vi "PrefDialog-old.vi"(8 "error in (no error)":errorcluster, 11 "MyPluginsBase in":refnum<class "NHRGridSim.lvclass">) -> (0 "error out":errorcluster, 1 "Save As":bool, 2 "Changed":bool, 3 "MyPluginsBase out":refnum<class "NHRGridSim.lvclass">)   [LabVIEW 2018, in "AcPwrPlugins.lvlib" / "NHRGridSim.lvclass"]
doc: "This VI opens up the modal preference dialog window and allows a user to configure the properties with new values, or keep the existing values from the last time the function was called. The user can also save the new values to a new file name and new type name using the save as button."
uses:
  NHRGridSim.lvclass
  C:/Program Files (x86)/National Instruments/LabVIEW 2018/user.lib/NIST/BaseClasses/BasePlugin_class/BasePlugin.lvclass
  C:/Users/Public/Projects/ICDAS/NistPluggableModules/AcPwr/AcPwrPlugins/AcPwrBaseClass/AcPwrBase.lvclass
  TypeDefs/Device(s)Settings.ctl
  TypeDefs/Modules.ctl
  Measurements.ctl
  TypeDefs/MeasurementType.ctl
  <userlib>/NIST/BaseClasses/BasePlugin_class/BasePlugin.lvclass/BasePlugin.ctl
  AcPwrBaseClass/AcPwrBase.lvclass/AcPwrBase.ctl
  <userlib>/NIST/BaseClasses/BasePlugin_class/Accessors/Read PluginIniFilePath.vi
  AcPwrBaseClass/Accessors/Read BaseConfig.vi
  AcPwrBaseClass/Accessors/Read BaseMeasurements.vi
  <userlib>/NIST/BaseClasses/BasePlugin_class/Accessors/Write PluginIniFilePath.vi
  <vilib>/Utility/config.llb/NI_LVConfig.lvlib
  AcPwrBaseClass/AcPwrBase.lvclass
panel:
  in  "Measurements":T1 {"Phase" items=["All", "A Phase", "B Phase", "C Phase"]}
  in  "Device(s)Settings":T3 {"Modules"."Phase (0: All)" items=["All", "A Phase", "B Phase", "C Phase"]; "Modules"."Mode" items=["3-Phase AC", "AC", "DC", "AC - AC - AC", "DC - DC - DC", "2-Phase AC - AC", "2-Phase AC - DC", "AC - AC", "AC - DC", "AC - AC - DC", "AC - DC - DC", "DC - AC", "DC - DC", "AC - DC - AC", "DC - AC - AC", "DC - AC - DC"]}
  in  "btnSaveAs":bool
  in  "Measurement RefreshTime (ms)":u32
  in  "btnSave":bool
  in  "btnCancel":bool
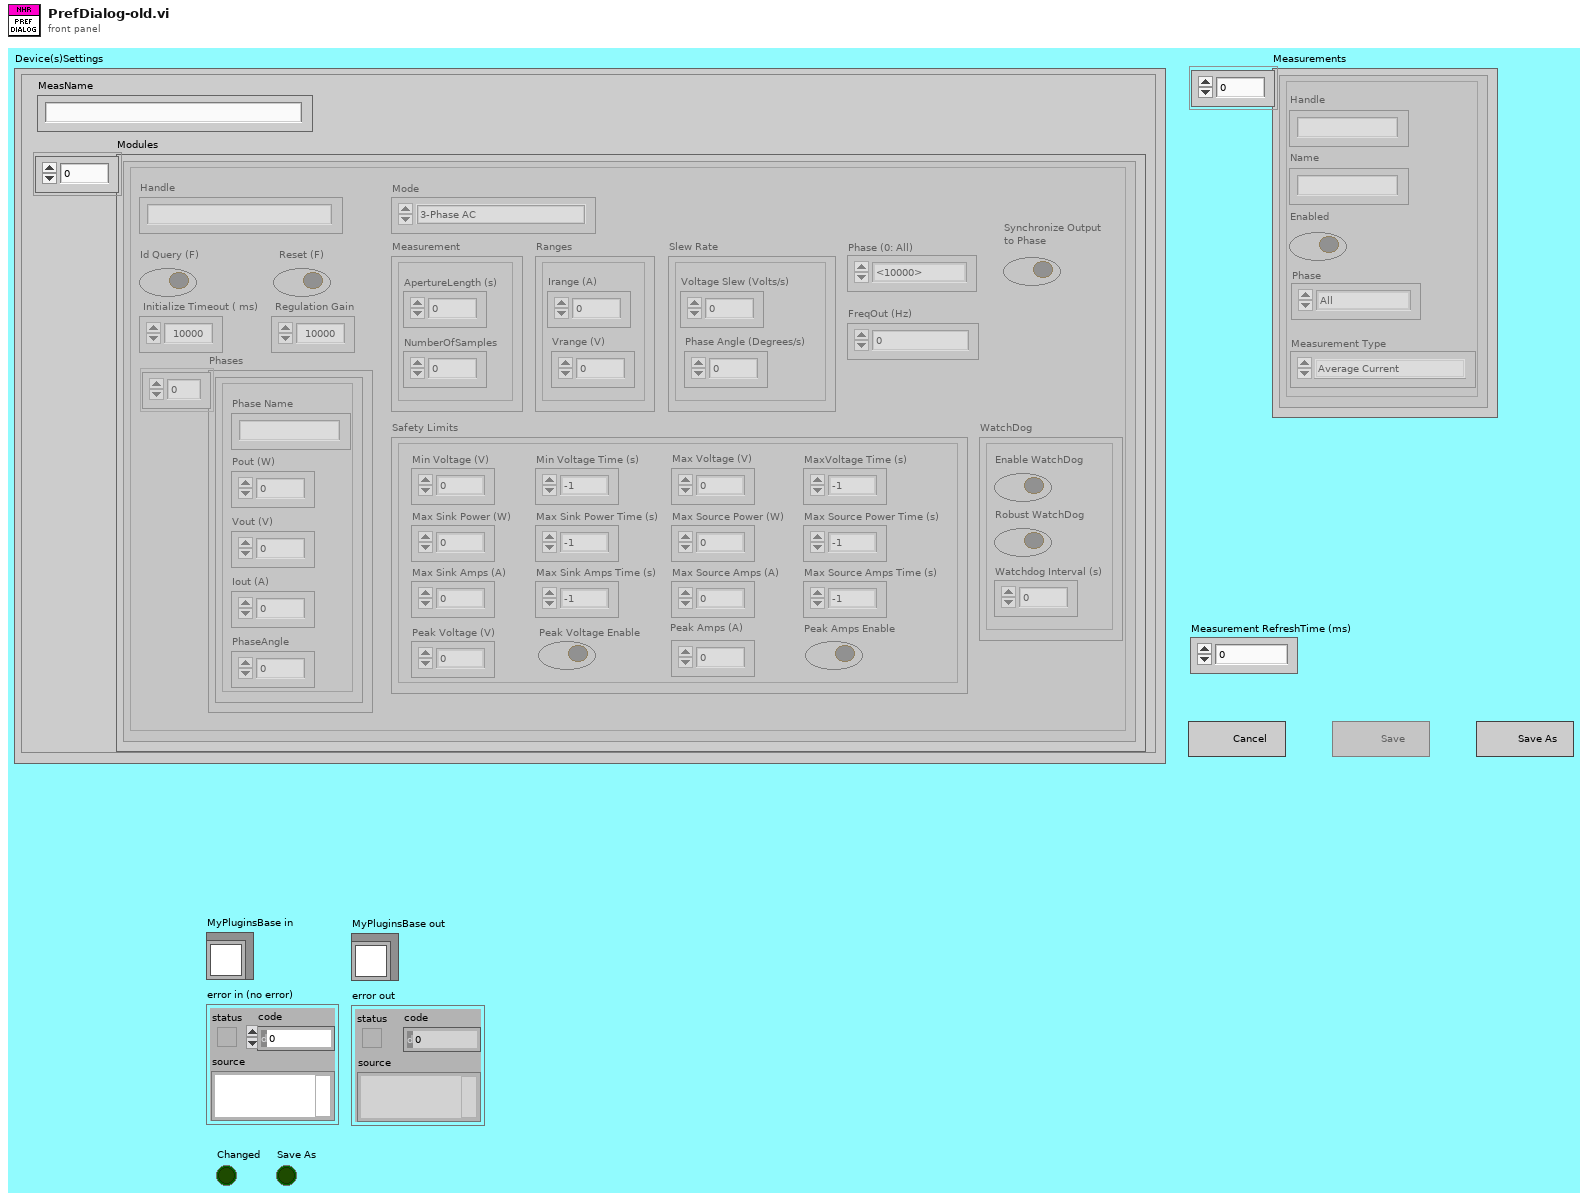
[diagram p1: front panel]
types:
  T1 = typedef "AcPwrPlugins.lvlib/NHRGridSim.lvclass/Measurements.ctl" = cluster{"Handle":string, "Name":string, "Enabled ":bool, "Measurement Value":dbl, "Phase ":i32, "Measurement Type ":T2}[]
  T2 = typedef "AcPwrPlugins.lvlib/NHRGridSim.lvclass/MeasurementType.ctl" = enum16{"Average Current", "Average Voltage"}
  T3 = typedef "AcPwrPlugins.lvlib/NHRGridSim.lvclass/Device(s)Settings.ctl" = cluster{"MeasName":string, "Modules":T4}
  T4 = typedef "AcPwrPlugins.lvlib/NHRGridSim.lvclass/Modules.ctl" = cluster{"Measurement":cluster{"ApertureLength (s)":dbl, "NumberOfSamples":u32}, "Ranges":cluster{"Irange (A)":dbl, "Vrange (V)":dbl}, "Mode":u8, "Handle":string, "FreqOut (Hz)":dbl, "Connected":bool, "btnIdQuery":bool, "btnReset":bool, "Initialize Timeout ( ms)":u32, "Phase (0: All)":i32, "WatchDog":cluster{"Enable WatchDog":bool, "Robust WatchDog":bool, "Watchdog Interval (s)":dbl}, "Safety Limits":cluster{"Min Voltage (V)":dbl, "Min Voltage Time (s)":dbl, "Max Voltage (V)":dbl, "MaxVoltage Time (s)":dbl, "Max Source Amps (A)":dbl, "Max Source Amps Time (s)":dbl, "Max Sink Amps (A)":dbl, "Max Sink Amps Time (s)":dbl, "Max Source Power (W)":dbl, "Max Source Power Time (s)":dbl, "Max Sink Power (W)":dbl, "Max Sink Power Time (s)":dbl, "Peak Voltage (V)":dbl, "Peak Voltage Enable":bool, "Peak Amps (A)":dbl, "Peak Amps Enable":bool}, "Phases":cluster{"Pout (W)":dbl, "Iout (A)":dbl, "PhaseAngle":dbl, "Vout (V)":dbl, "Phase Name":string}[], "Regulation Gain":dbl, "ChangeOntheFly":bool, "Synchronize Output \nto Phase":bool, "Slew Rate":cluster{"Voltage Slew (Volts/s)":dbl, "Phase Angle (Degrees/s)":dbl}}[]
  T5 = enum32{"Invalid", "Standard", "Closed", "Hidden", "Minimized", "Maximized"}
  T6 = enum32{"Invalid", "Default", "Floating", "Floating/Auto-Hide", "Modal"}
  T7 = enum8{"Enabled", "Disabled", "Disabled and Grayed Out"}
  T8 = cluster{"Pout (W)":dbl, "Iout (A)":dbl, "PhaseAngle":dbl, "Vout (V)":dbl, "Phase Name":string}[]
  T9 = cluster{"Pout (W)":dbl, "Iout (A)":dbl, "PhaseAngle":dbl, "Vout (V)":dbl, "Phase Name":string}
  T10 = cluster{"Measurement":cluster{"ApertureLength (s)":dbl, "NumberOfSamples":u32}, "Ranges":cluster{"Irange (A)":dbl, "Vrange (V)":dbl}, "Mode":u8, "Handle":string, "FreqOut (Hz)":dbl, "Connected":bool, "btnIdQuery":bool, "btnReset":bool, "Initialize Timeout ( ms)":u32, "Phase (0: All)":i32, "WatchDog":cluster{"Enable WatchDog":bool, "Robust WatchDog":bool, "Watchdog Interval (s)":dbl}, "Safety Limits":cluster{"Min Voltage (V)":dbl, "Min Voltage Time (s)":dbl, "Max Voltage (V)":dbl, "MaxVoltage Time (s)":dbl, "Max Source Amps (A)":dbl, "Max Source Amps Time (s)":dbl, "Max Sink Amps (A)":dbl, "Max Sink Amps Time (s)":dbl, "Max Source Power (W)":dbl, "Max Source Power Time (s)":dbl, "Max Sink Power (W)":dbl, "Max Sink Power Time (s)":dbl, "Peak Voltage (V)":dbl, "Peak Voltage Enable":bool, "Peak Amps (A)":dbl, "Peak Amps Enable":bool}, "Phases":cluster{"Pout (W)":dbl, "Iout (A)":dbl, "PhaseAngle":dbl, "Vout (V)":dbl, "Phase Name":string}[], "Regulation Gain":dbl, "ChangeOntheFly":bool, "Synchronize Output \nto Phase":bool, "Slew Rate":cluster{"Voltage Slew (Volts/s)":dbl, "Phase Angle (Degrees/s)":dbl}}
  T11 = typedef "AcPwrPlugins.lvlib/AcPwrBase.lvclass/BaseConfig.ctl" = cluster{"Frequency":dbl, "FrequencyRange":dbl[], "Phases":T12[], "Name":string, "PluginConfigVariant":variant, "PluginMeasVariant":variant}
  T12 = typedef "AcPwrPlugins.lvlib/AcPwrBase.lvclass/Phase.ctl" = cluster{"Name":string, "Enabled":bool, "VoltageLevel":dbl, "Handle":string, "VoltageRange":dbl[], "Connected":bool, "CurrentLimit":dbl, "Waveform":string}
  T13 = typedef "AcPwrPlugins.lvlib/AcPwrBase.lvclass/BaseMeasurements.ctl" = cluster{"Handle":string, "Name":string, "Enabled":bool, "Measurement Value":dbl, "btnMeasFetch":bool, "Chroma Hold Peak Current Measurement":bool, "Chroma Measurement Type":T14, "Chroma Protection Status String":string, "NHRDC Fetch Method":i32, "NHRDC Fetch Time (s)":sgl, "NHRDC Measurement Type":i32, "NHRGridSim Measurement Type ":enum16{"Average Current", "Max Current", "Min Current", "Average Voltage", "Max Voltage", "Min Voltage", "Average True Power", "Max True Power", "Min True Power", "Average Apparent Power", "Max Apparent Power", "Min Apparent Power", "Power Factor", "Crest Factor"}, "NHRGridSim Phase ":i32, "PPS Measurement Type ":enum16{"Voltage RMS L-N", "Voltage RMS L-L", "Frequency", "Current RMS", "Current Peak", "Crest Factor", "Power Factor", "Power VA", "Real Power"}, "PPS Channel Name":enum16{"A", "B", "C"}}[]
  T14 = typedef "AcPwrPlugins.lvlib/ChromaAcLoad.lvclass/MeasurementType.ctl" = enum16{"Voltage (Vrms or V)", "Current (Arms or A)", "Power (W)", "Peak Voltage (V)", "Peak Current (A)", "Peak Power (W)", "Frequency (Hz)", "Resistance (Ohms)", "Voltage Overshoot (V)", "Positive Peak Current (A)", "Voltage Undershoot (V)", "Negative Peak Current (A)", "Apparent Power (VA)", "Reacitive Power (VAR)", "Voltage THD", "Power Factor", "Current's Crest Factor"}
  T15 = typedef "NI_LVConfig.lvlib/Config Data RefNum.ctl" = refnum<k1>
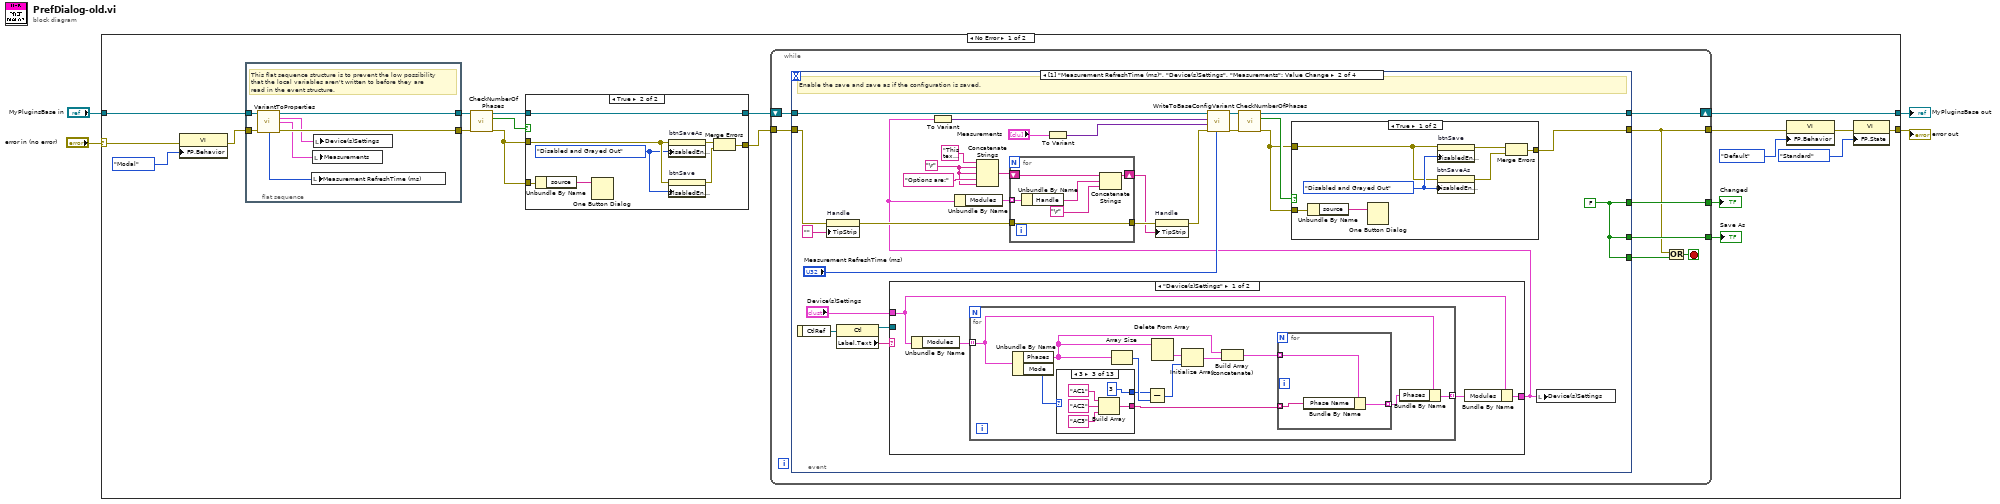
[diagram p0: block diagram]
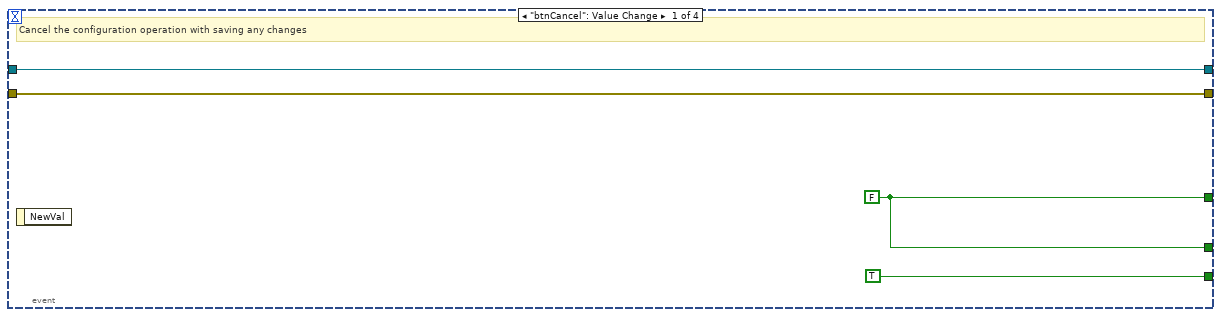
[diagram p2: hidden frame]
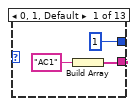
[diagram p3: hidden frame]
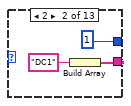
[diagram p4: hidden frame]
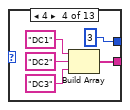
[diagram p5: hidden frame]
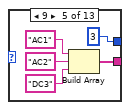
[diagram p6: hidden frame]
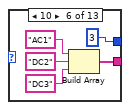
[diagram p7: hidden frame]
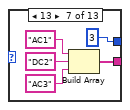
[diagram p8: hidden frame]
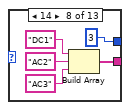
[diagram p9: hidden frame]
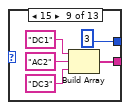
[diagram p10: hidden frame]
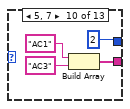
[diagram p11: hidden frame]
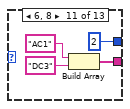
[diagram p12: hidden frame]
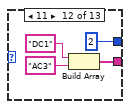
[diagram p13: hidden frame]
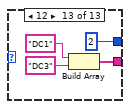
[diagram p14: hidden frame]
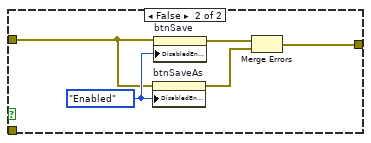
[diagram p16: hidden frame]
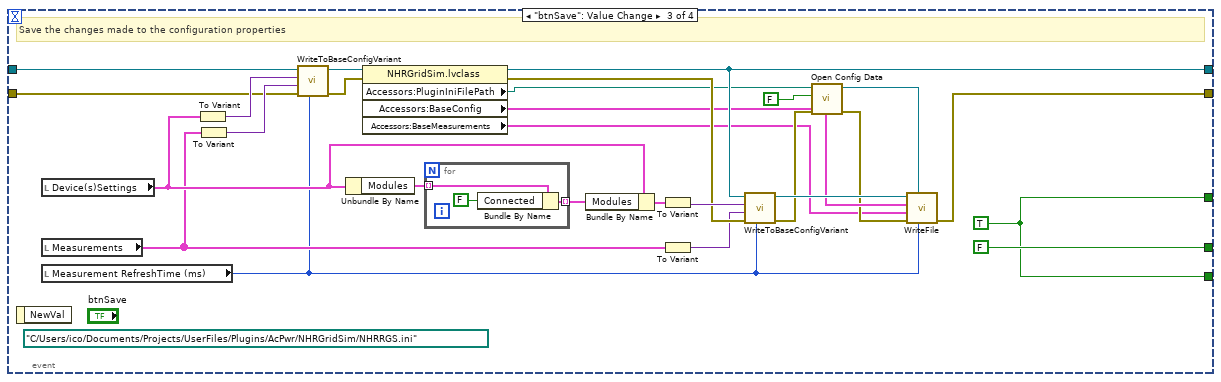
[diagram p17: hidden frame]
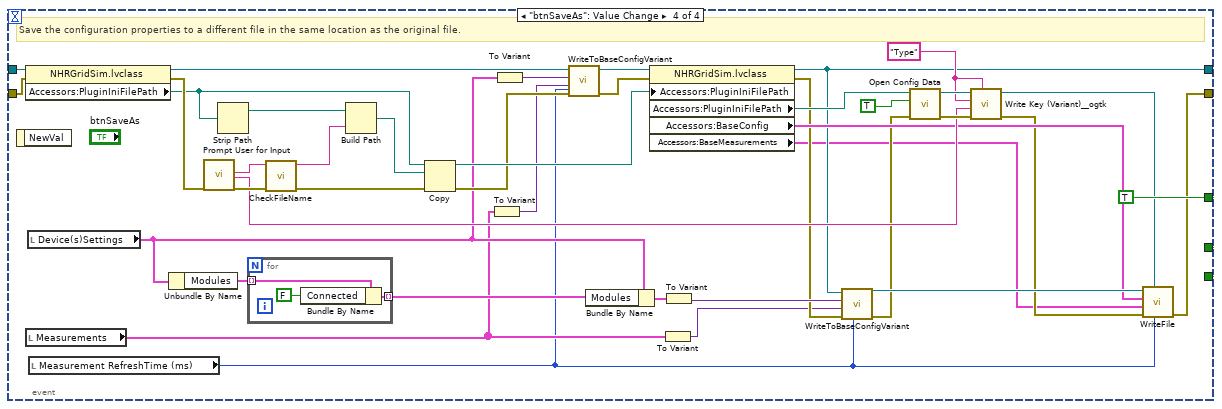
[diagram p18: hidden frame]
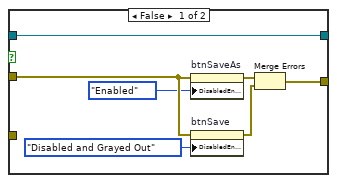
[diagram p19: hidden frame]
diagram:
  n1 = case shown="No Error" "error in (no error)" {
    selector: "error in (no error)" -> [w21 w256]
    tunnel: "MyPluginsBase in" -> [w16 w255]
    tunnel: [w14 w255] -> w2
    tunnel: [w12 w256] -> w1
    frame No Error {
      n2 = property class="VI"(error in=w21, "FP.Behavior"=T6."Modal" ("Front Panel Window:Behavior")) -> (error out=w17:errorcluster)  [unwired: 1 in, 1 out]
      n3 = flat-sequence {
        tunnel: w16 -> [w30]
        tunnel: [w29] -> w9
        tunnel: [w27] -> w10
        tunnel: w17 -> [w28]
        frame #0 {
          # "This flat sequence structure is to prevent the low possibility that the local variables aren't written to before they are read in the event structure."
          n4 = call "VariantToProperties.vi"("NHRGridSim in"=w30, "error in (no error)"=w28) -> ("NHRGridSim out"=w29:refnum<class "NHRGridSim.lvclass">, "Device(s)Settings"=w26:T3, "Measurements"=w24:T1, "Measurement Refresh Time (ms)"=w25:u32, "error out"=w27:errorcluster)  [unwired: 7 in, 2 out]
          n5 = local write "Measurement RefreshTime (ms)"(w25) -> ()
          n6 = local write "Measurements"(w24) -> ()
          n7 = local write "Device(s)Settings"(w26) -> ()
        }
      }
      n8 = call "CheckNumberOfPhases.vi"("error in (no error)"=w10, "NHRGridSim in"=w9) -> ("error out"=w7:errorcluster, "Boolean"=w8:bool, "NHRGridSim out"=w6:refnum<class "NHRGridSim.lvclass">)  [unwired: 6 in, 1 out]
      n9 = case shown="True" w8 {
        tunnel: w7 -> [w245 w253]
        tunnel: [w244 w252] -> w15
        tunnel: w7 -> [_ w249]
        tunnel: w6 -> [w240 w247]
        tunnel: [w240 w247] -> w5
        frame False {
          # "Check if the number of Phases=Loads. If no disables the ability\nto save as."
          n10 = property on="btnSaveAs" class="Bool"(error in=w245, "DisabledEnum"=T7."Enabled" ("Disabled")) -> (error out=w246:errorcluster)  [unwired: 1 in, 1 out]
          n11 = property on="btnSave" class="Bool"(error in=w245, "DisabledEnum"=T7."Disabled and Grayed Out" ("Disabled")) -> (error out=w243:errorcluster)  [unwired: 1 in, 1 out]
          n12 = Merge Errors(w246, w243) -> (w244:errorcluster)
        }
        frame True {
          w250 = T7."Disabled and Grayed Out" ("Disabled")
          # "Check if the number of Phases=Loads. If no disables the ability\nto save as."
          n13 = Unbundle By Name(w249) -> ("source"=w248:string)
          n14 = One Button Dialog(message=w248) -> ()  [unwired: 1 in, 1 out]
          n15 = property on="btnSaveAs" class="Bool"(error in=w253, "DisabledEnum"=w250) -> (error out=w254:errorcluster)  [unwired: 1 in, 1 out]
          n16 = property on="btnSave" class="Bool"(error in=w253, "DisabledEnum"=w250) -> (error out=w251:errorcluster)  [unwired: 1 in, 1 out]
          n17 = Merge Errors(w254, w251) -> (w252:errorcluster)
        }
      }
      n18 = while {
        shift-right: [w36] -> w14
        shift-left: w5 -> [w37]
        tunnel: [w38] -> w22
        tunnel: [w34] -> w13
        tunnel: w15 -> [w35]
        tunnel: [w31] -> w11
        stop <- w33 stop-if-true
        n19 = event shown="[1] \"Measurement RefreshTime (ms)\", \"Device(s)Settings\", \"Measurements\": Value Change" {
          selector: _ -> [_ _ _ _]
          dyn-events: _ -> [_ _ _ _]
          timeout: _ -> [_ _ _ _]
          tunnel: [w39 w69 w190 w231] -> w38
          tunnel: [TRUE w69 w190 w231] -> w32
          tunnel: w37 -> [w41 w61 w171 w225]
          tunnel: [w41 w64 w185 w209] -> w36
          tunnel: [w40 w70 w187 w211] -> w31
          tunnel: w35 -> [w40 w55 w168 w224]
          tunnel: [w39 w69 FALSE w231] -> w34
          event "btnCancel": Value Change {
            w39 = FALSE
            # "Cancel the configuration operation with saving any changes"
            n20 = event-data() -> ()  [unwired: 1 in, 1 out]
          }
          event "Measurement RefreshTime (ms)": Value Change {
            w66 = "\r"
            w69 = FALSE
            # "Enable the save and save as if the configuration is saved."
            n21 = event-data() -> ("CtlRef"=w47:refnum<vi>)  [unwired: 1 in]
            n22 = property on="Handle" class="Str"(error in=w55, "TipStrip"="" ("Tip Strip")) -> (error out=w54:errorcluster)  [unwired: 1 in, 1 out]
            n23 = property class="Ctl"(reference=w47) -> (reference out=w45:refnum<vi>, "Label.Text"=w46:string)  [unwired: 1 in, 1 out]
            n24 = case shown="\"Device(s)Settings\"" w46 {
              tunnel: "Device(s)Settings" -> [w73 w147]
              tunnel: w45 -> [_ _]
              tunnel: [w71 w147] -> w44
              frame "Device(s)Settings" {
                n25 = Unbundle By Name(w73) -> ("Modules"=w74:T4)
                n26 = for {
                  tunnel: w74 -> [w84] mode=indexing
                  tunnel: [w83] -> w72 mode=indexing
                  n27 = Unbundle By Name(w84) -> ("Phases"=w79:T8, "Mode"=w86:u8)
                  n28 = case shown="3" w86 {
                    tunnel: [w91 w94 w99 w104 w109 w114 w119 w124 w129 w133 w137 w141 w145] -> w81
                    tunnel: [1 1 3 3 3 3 3 3 3 2 2 2 2] -> w82
                    frame 0, 1, Default {
                      n29 = Build Array("AC1") -> (w91:string[])
                    }
                    frame 2 {
                      n30 = Build Array("DC1") -> (w94:string[])
                    }
                    frame 3 {
                      n31 = Build Array("AC1", "AC2", "AC3") -> (w99:string[])
                    }
                    frame 4 {
                      n32 = Build Array("DC1", "DC2", "DC3") -> (w104:string[])
                    }
                    frame 9 {
                      n33 = Build Array("AC1", "AC2", "DC3") -> (w109:string[])
                    }
                    frame 10 {
                      n34 = Build Array("AC1", "DC2", "DC3") -> (w114:string[])
                    }
                    frame 13 {
                      n35 = Build Array("AC1", "DC2", "AC3") -> (w119:string[])
                    }
                    frame 14 {
                      n36 = Build Array("DC1", "AC2", "AC3") -> (w124:string[])
                    }
                    frame 15 {
                      n37 = Build Array("DC1", "AC2", "DC3") -> (w129:string[])
                    }
                    frame 5, 7 {
                      n38 = Build Array("AC1", "AC3") -> (w133:string[])
                    }
                    frame 6, 8 {
                      n39 = Build Array("AC1", "DC3") -> (w137:string[])
                    }
                    frame 11 {
                      n40 = Build Array("DC1", "AC3") -> (w141:string[])
                    }
                    frame 12 {
                      n41 = Build Array("DC1", "DC3") -> (w145:string[])
                    }
                  }
                  n42 = Array Size(array=w79) -> (size(s)=w85:i32)
                  n43 = Subtract(x=w82, y=w85) -> (x-y=w76:i32)
                  n44 = Delete From Array(array=w79) -> (deleted portion=w77:T9)  [unwired: 2 in, 1 out]
                  n45 = Initialize Array(w77, w76) -> (w78:T8)
                  n46 = Build Array (concatenate)(w79, w78) -> (w80:T8)
                  n47 = for {
                    tunnel: w80 -> [w89] mode=indexing
                    tunnel: w81 -> [w87] mode=indexing
                    tunnel: [w88] -> w75 mode=indexing
                    n48 = Bundle By Name(cluster=w89, "Phase Name"=w87) -> (w88:T9)
                  }
                  n49 = Bundle By Name(cluster=w84, "Phases"=w75) -> (w83:T10)
                }
                n50 = Bundle By Name(cluster=w73, "Modules"=w72) -> (w71:T3)
              }
              frame Default {
              }
            }
            n51 = To Variant(anything=w44) -> (Variant=w62:variant)
            n52 = Unbundle By Name(w44) -> ("Modules"=w57:T4)
            n53 = Concatenate Strings("This text in this handle of the instrument and entered in the  \nhandle control in the Phases array EXACTLY, lest the attempt \nto interact with the instrument will fail.", w66, w66, "Options are:" ("Handle"), w66) -> (w65:string)
            n54 = for {
              shift-right: [w153] -> w51
              shift-left: w65 -> [w152]
              tunnel: w57 -> [w151] mode=indexing
              tunnel: w54 -> [w148]
              tunnel: [w148] -> w52
              n55 = Unbundle By Name(w151) -> ("Handle"=w150:string)
              n56 = Concatenate Strings(w152, w150, "\r") -> (w153:string)
            }
            n57 = To Variant(anything="Measurements") -> (Variant=w48:variant)
            n58 = property on="Handle" class="Str"(error in=w52, "TipStrip"=w51) -> (error out=w53:errorcluster)  [unwired: 1 in, 1 out]
            n59 = call "WriteToBaseConfigVariant.vi"("Measurement RefreshTime (ms)"="Measurement RefreshTime (ms)", "error in (no error)"=w53, "Meas"=w48, "Config"=w62, "NHRGridSim in"=w61) -> ("error out"=w59:errorcluster, "NHRGridSim out"=w60:refnum<class "NHRGridSim.lvclass">)  [unwired: 5 in]
            n60 = call "CheckNumberOfPhases.vi"("error in (no error)"=w59, "NHRGridSim in"=w60) -> ("error out"=w58:errorcluster, "Boolean"=w63:bool, "NHRGridSim out"=w64:refnum<class "NHRGridSim.lvclass">)  [unwired: 6 in, 1 out]
            n61 = case shown="True" w63 {
              tunnel: w58 -> [w157 w162]
              tunnel: [w156 w161] -> w70
              tunnel: w58 -> [w154 _]
              frame True {
                w158 = T7."Disabled and Grayed Out" ("Disabled")
                n62 = Unbundle By Name(w154) -> ("source"=w155:string)
                n63 = One Button Dialog(message=w155) -> ()  [unwired: 1 in, 1 out]
                n64 = property on="btnSaveAs" class="Bool"(error in=w157, "DisabledEnum"=w158) -> (error out=w160:errorcluster)  [unwired: 1 in, 1 out]
                n65 = property on="btnSave" class="Bool"(error in=w157, "DisabledEnum"=w158) -> (error out=w159:errorcluster)  [unwired: 1 in, 1 out]
                n66 = Merge Errors(w159, w160) -> (w156:errorcluster)
              }
              frame False {
                w163 = T7."Enabled" ("Disabled")
                n67 = property on="btnSaveAs" class="Bool"(error in=w162, "DisabledEnum"=w163) -> (error out=w165:errorcluster)  [unwired: 1 in, 1 out]
                n68 = property on="btnSave" class="Bool"(error in=w162, "DisabledEnum"=w163) -> (error out=w164:errorcluster)  [unwired: 1 in, 1 out]
                n69 = Merge Errors(w164, w165) -> (w161:errorcluster)
              }
            }
            n70 = local write "Device(s)Settings"(w44) -> ()
          }
          event "btnSave": Value Change {
            (unwired) path "C:/Users/ico/Documents/Projects/UserFiles/Plugins/AcPwr/NHRGridSim/NHRRGS.ini" ("Accessors:PluginIniFilePath")
            w190 = TRUE ("StartMeas")
            # "Save the changes made to the configuration properties"
            n71 = event-data() -> ()  [unwired: 1 in, 1 out]
            n72 = local read "Device(s)Settings"() -> (w170:T3)
            n73 = local read "Measurements"() -> (w169:T1)
            n74 = local read "Measurement RefreshTime (ms)"() -> (w167:u32)
            n75 = To Variant(anything=w170) -> (Variant=w175:variant)
            n76 = To Variant(anything=w169) -> (Variant=w174:variant)
            n77 = call "WriteToBaseConfigVariant.vi"("Measurement RefreshTime (ms)"=w167, "error in (no error)"=w168, "Meas"=w174, "Config"=w175, "NHRGridSim in"=w171) -> ("error out"=w172:errorcluster, "NHRGridSim out"=w173:refnum<class "NHRGridSim.lvclass">)  [unwired: 5 in]
            n78 = Unbundle By Name(w170) -> ("Modules"=w188:T4)
            n79 = property class="NHRGridSim.lvclass"(reference=w173, error in=w172) -> (reference out=w185:refnum<class "NHRGridSim.lvclass">, error out=w182:errorcluster, "Accessors:PluginIniFilePath"=w166:path, "Accessors:BaseConfig"=w181:T11, "Accessors:BaseMeasurements"=w178:T13)
            n80 = for {
              tunnel: w188 -> [w195] mode=indexing
              tunnel: [w194] -> w189 mode=indexing
              n81 = Bundle By Name(cluster=w195, "Connected"=FALSE) -> (w194:T10)
            }
            n82 = Bundle By Name(cluster=w170, "Modules"=w189) -> (w177:T3)
            n83 = To Variant(anything=w177) -> (Variant=w186:variant)
            n84 = To Variant(anything=w169) -> (Variant=w176:variant)
            n85 = call "WriteToBaseConfigVariant.vi"("Measurement RefreshTime (ms)"=w167, "error in (no error)"=w182, "Meas"=w176, "Config"=w186, "NHRGridSim in"=w185) -> ("error out"=w183:errorcluster, "NHRGridSim out"=w184:refnum<class "NHRGridSim.lvclass">)  [unwired: 5 in]
            n86 = call <vilib>:"Open Config Data.vi"("error in (no error)"=w183, "create file if necessary (T)"=FALSE, "configuration file path"=w166) -> ("error out"=w179:errorcluster, "refnum"=w180:T15)  [unwired: 6 in, 1 out]
            n87 = call-dynamic "WriteFile.vi"("RefreshTime"=w167, "Refnum in"=w180, "error in (no error)"=w179, "BaseMeasurements"=w178, "BaseConfiguration"=w181, "NHRGridSim in"=w184) -> ("error out"=w187:errorcluster)  [unwired: 4 in, 1 out]
          }
          event "btnSaveAs": Value Change {
            w226 = "Type" ("section (optional)")
            w231 = TRUE
            # "Save the configuration properties to a different file in the same location as the original file."
            n88 = event-data() -> ()  [unwired: 1 in, 1 out]
            n89 = property class="NHRGridSim.lvclass"(reference=w225, error in=w224) -> (reference out=w201:refnum<class "NHRGridSim.lvclass">, error out=w223:errorcluster, "Accessors:PluginIniFilePath"=w222:path)
            n90 = local read "Measurements"() -> (w198:T1)
            n91 = local read "Device(s)Settings"() -> (w199:T3)
            n92 = local read "Measurement RefreshTime (ms)"() -> (w196:u32)
            n93 = Unbundle By Name(w199) -> ("Modules"=w219:T4)
            n94 = call "Prompt User for Input"("error in (no error)"=w223) -> ("File Name"=w221:string, "PluginType"=w227:string, "error out"=w228:errorcluster)  [unwired: 15 in, 1 out]
            n95 = Strip Path(path=w222) -> (stripped path=w233:path)  [unwired: 1 out]
            n96 = for {
              tunnel: w219 -> [w239] mode=indexing
              tunnel: [w238] -> w220 mode=indexing
              n97 = Bundle By Name(cluster=w239, "Connected"=FALSE) -> (w238:T10)
            }
            n98 = call "CheckFileName.vi"("Error In"=w228, "File Name in"=w221) -> ("Error Out"=w229:errorcluster, "File Name out"=w230:string)  [unwired: 8 in]
            n99 = Build Path(base path=w233, name or relative path=w230) -> (appended path=w232:path)
            n100 = Copy(8:w229, 10:w232, 11:w222) -> (0:w204:errorcluster, 3:w215:path)  [unwired: 2 in, 1 out]
            n101 = To Variant(anything=w198) -> (Variant=w197:variant)
            n102 = To Variant(anything=w199) -> (Variant=w200:variant)
            n103 = call "WriteToBaseConfigVariant.vi"("Measurement RefreshTime (ms)"=w196, "error in (no error)"=w204, "Meas"=w197, "Config"=w200, "NHRGridSim in"=w201) -> ("error out"=w203:errorcluster, "NHRGridSim out"=w202:refnum<class "NHRGridSim.lvclass">)  [unwired: 5 in]
            n104 = Bundle By Name(cluster=w199, "Modules"=w220) -> (w218:T3)
            n105 = property class="NHRGridSim.lvclass"(reference=w202, error in=w203, "Accessors:PluginIniFilePath"=w215) -> (reference out=w209:refnum<class "NHRGridSim.lvclass">, error out=w210:errorcluster, "Accessors:PluginIniFilePath"=w214:path, "Accessors:BaseConfig"=w213:T11, "Accessors:BaseMeasurements"=w206:T13)
            n106 = To Variant(anything=w198) -> (Variant=w205:variant)
            n107 = To Variant(anything=w218) -> (Variant=w217:variant)
            n108 = call "WriteToBaseConfigVariant.vi"("Measurement RefreshTime (ms)"=w196, "error in (no error)"=w210, "Meas"=w205, "Config"=w217, "NHRGridSim in"=w209) -> ("error out"=w208:errorcluster, "NHRGridSim out"=w216:refnum<class "NHRGridSim.lvclass">)  [unwired: 5 in]
            n109 = call <vilib>:"Open Config Data.vi"("error in (no error)"=w208, "create file if necessary (T)"=TRUE, "configuration file path"=w214) -> ("error out"=w235:errorcluster, "refnum"=w234:T15)  [unwired: 6 in, 1 out]
            n110 = call <userlib>:"Write Key (Variant)__ogtk.vi"("section"=w226, "error in (no error)"=w235, "key-value"=w227, "key (optional)"=w226, "refnum"=w234) -> ("error out"=w207:errorcluster, "refnum out"=w212:T15)  [unwired: 5 in]
            n111 = call-dynamic "WriteFile.vi"("RefreshTime"=w196, "Refnum in"=w212, "error in (no error)"=w207, "BaseMeasurements"=w206, "BaseConfiguration"=w213, "NHRGridSim in"=w216) -> ("error out"=w211:errorcluster)  [unwired: 4 in, 1 out]
          }
        }
        n112 = Or(x=w31, y=w32) -> (x .or. y?=w33:bool)
      }
      "Changed" <- w22
      "Save As" <- w13
      n113 = property class="VI"(error in=w11, "FP.Behavior"=T6."Default" ("Front Panel Window:Behavior")) -> (error out=w20:errorcluster)  [unwired: 1 in, 1 out]
      n114 = property class="VI"(error in=w20, "FP.State"=T5."Standard" ("Front Panel Window:State")) -> (error out=w12:errorcluster)  [unwired: 1 in, 1 out]
    }
    frame Error {
    }
  }
  "MyPluginsBase out" <- w2
  "error out" <- w1
